vi "Search With Pattern.vi"(10 "Regular Expression":string, 11 "Array":string[](array[string])) -> (2 "Numeric":i32)   [LabVIEW 2017, in "CSM-Helper.lvclass"]
doc: "### Search With Pattern.vi\n\n-- <b>Controls</b> --\n- <b>regular expression</b>:\n- <b>Array</b>:\n\n-- <b>Indicators</b> --\n- <b>Numeric</b>:"
uses:
  CSM-Helper.lvclass
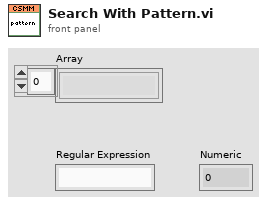
[diagram p1: front panel]
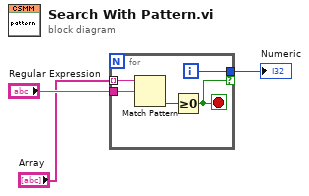
[diagram p0: block diagram]
diagram:
  n1 = for {
    tunnel: "Array" -> [w8] mode=indexing
    tunnel: "Regular Expression" -> [w7]
    tunnel: [w5] -> w3 if=w4
    i -> [w5]
    stop <- w4 stop-if-true
    n2 = Match Pattern(string=w8, regular expression=w7) -> (offset past match=w6:i32)  [unwired: 1 in, 3 out]
    n3 = Greater Or Equal To 0?(x=w6) -> (x >= 0?=w4:bool)
  }
  "Numeric" <- w3
